vi "AD5781SetVolt.vi"(3 "Send":bool=TRUE, 5 "SetVolt":u32 format="%032b") -> (0 "Readback":u32 format="%024b", 1 "Readback 0":u32 format="%032b", 2 "timedOut":bool)   [LabVIEW 2014]
uses:
  <vilib>/rvi/Emulation/niFpgaGetClockAttributes.vi
  <vilib>/rvi/Emulation/niFpgaSctlEmulationGetInTimedLoop.vi
  <vilib>/rvi/Emulation/niFpgaEmulationReportErrorSimple.vi
  <vilib>/rvi/eio/common/nirviEmuTemplateMethod_errors.vi
  <vilib>/rvi/Emulation/niFpgaCriticalErrorInLSC.vi
  Code/FPGA SPI_Globals.vi
  <vilib>/rvi/Emulation/niFpgaProcessEmulError.vi
  <vilib>/eio/EIONode/EIONode.xnode
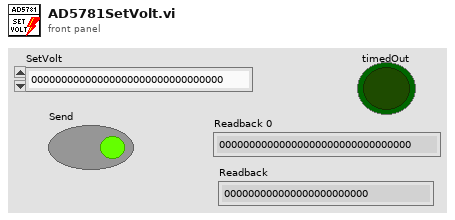
[diagram p1: front panel]
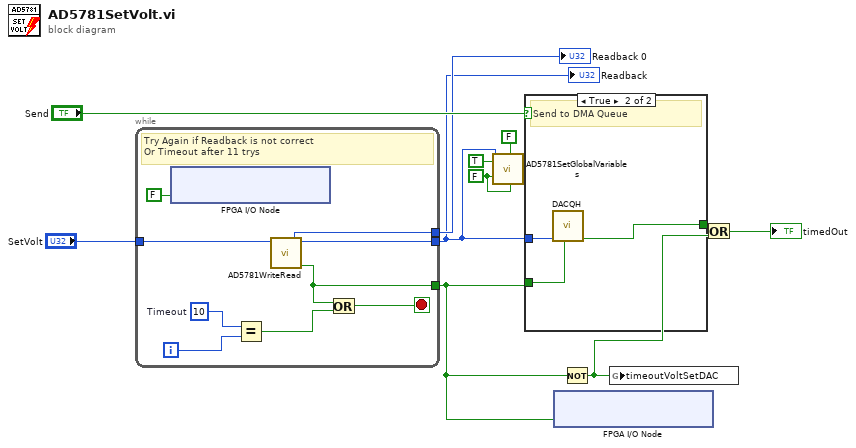
[diagram p0: block diagram]
diagram:
  w2 = FALSE ("write setDACRegister")
  n1 = while {
    tunnel: "SetVolt" -> [w20]
    tunnel: [w15] -> w4
    tunnel: [w14] -> w9
    tunnel: [w12] -> w8
    i -> [w19]
    stop <- w17 stop-if-true
    w18 = 10  # Timeout
    # "Try Again if Readback is not correct\nOr Timeout after 11 trys"
    n2 = xnode "FPGA I/O Node"("voltSetFlagDio10Con1"=FALSE) -> ()  [unwired: 1 in, 1 out]
    n3 = Equal?(x=w18, y=w19) -> (x = y?=w16:bool)
    n4 = call "AD5781WriteRead.vi"("Write"=w20) -> ("WriteEqualsRead"=w14:bool, "Readback 0"=w12:u32, "Readback"=w15:u32)  [unwired: 5 in]
    n5 = Or(x=w14, y=w16) -> (x .or. y?=w17:bool)
  }
  "Readback" <- w4
  "Readback 0" <- w8
  n6 = call "AD5781SetGlobalVariables.vi"("actDACRegister"=w4, "write actDACRegister"=TRUE, "write setDACRegister"=w2, "write DacStateCmdByHost"=FALSE, "write DacState"=w2) -> ()  [unwired: 15 in]
  n7 = case shown="True" "Send" {
    tunnel: w4 -> [_ w21]
    tunnel: w9 -> [_ w23]
    tunnel: [_ w22] -> w5
    frame False {
    }
    frame True {
      # "Send to DMA Queue"
      n8 = call "DACQH.vi"("writeEqualsRead?"=w23, "Readback"=w21) -> ("DACQuWriteTimeout"=w22:bool)  [unwired: 9 in]
    }
  }
  n9 = xnode "FPGA I/O Node"("voltSetFlagDio10Con1"=w9) -> ()  [unwired: 1 in, 1 out]
  n10 = Not(x=w9) -> (.not. x?=w7:bool)
  n11 = global write "FPGA SPI_Globals.vi" "timeoutVoltSetDAC"(w7) -> ()
  n12 = Or(x=w5, y=w7) -> (x .or. y?=→"timedOut":bool)
